vi "LogError.vi"(8 "error in":errorcluster) -> (0 "error out":errorcluster)   [LabVIEW 2014, in "Error Logger.lvclass"]
uses:
  Error Logger.lvclass
  Controls/Error Data.ctl
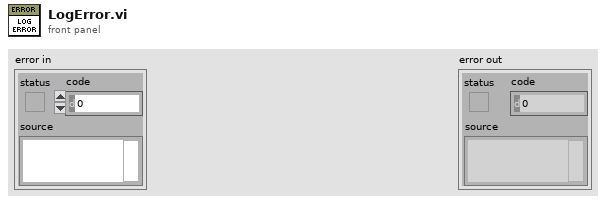
[diagram p1: front panel]
types:
  T1 = typedef "Error Logger.lvclass/Error Data.ctl" = cluster{"Message Type":enum16{"Information", "Warning", "Error"}, "Code":string, "Source":string}
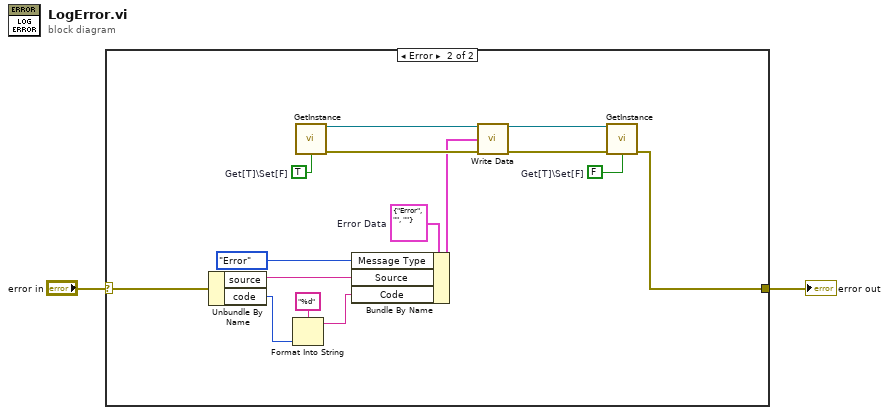
[diagram p0: block diagram]
diagram:
  n1 = case shown="Error" "error in" {
    selector: "error in" -> [w3 w15]
    tunnel: [w3 w12] -> w1
    frame No Error {
    }
    frame Error {
      w4 = FALSE  # Get[T]\Set[F]
      w11 = T1 {"Message Type"=enum."Error", "Code"="", "Source"=""}  # Error Data
      w18 = TRUE  # Get[T]\Set[F]
      n2 = Unbundle By Name(w15) -> ("source"=w9:string, "code"=w6:i32)
      n3 = Format Into String(format string="%d", w6) -> (resulting string=w7:string)  [unwired: 2 in, 1 out]
      n4 = call "GetInstance.vi"("Get[T]\\Set[F]"=w18) -> ("Error Logger out"=w17:refnum<class "Error Logger.lvclass">, "error out"=w16:errorcluster)  [unwired: 13 in]
      n5 = Bundle By Name(cluster=w11, "Message Type"=enum16{"Information", "Warning", "Error"}."Error", "Source"=w9, "Code"=w7) -> (w8:T1)
      n6 = call "Write Data.vi"("Error Logger in"=w17, "Error Data"=w8, "error in (no error)"=w16) -> ("Error Logger out"=w13:refnum<class "Error Logger.lvclass">, "error out"=w14:errorcluster)  [unwired: 11 in]
      n7 = call "GetInstance.vi"("Error Logger in"=w13, "error in (no error)"=w14, "Get[T]\\Set[F]"=w4) -> ("error out"=w12:errorcluster)  [unwired: 11 in, 1 out]
    }
  }
  "error out" <- w1
